vi "prep.vi"(8 "error in (no error)":errorcluster, 9 "Coordinate System":enum16{"Cartesian", "Cylindrical", "Spherical"}(ring), 10 "Plot processed data In":T1 caption="Data In", 11 "Parametric in":refnum<class "Parametric.lvclass">) -> (0 "error out":errorcluster, 2 "Plot Processed Data Out":T1 caption="Data Out", 3 "Parametric out":refnum<class "Parametric.lvclass">)   [LabVIEW 2017, in "Parametric.lvclass"]
uses:
  <vilib>/Native 3D Graph/classes/Parametric/Parametric.lvclass
  <vilib>/Native 3D Graph/xcontrol/Processed Data.ctl
  <vilib>/Native 3D Graph/typedefs/plot_rep_array.ctl
  <vilib>/Native 3D Graph/typedefs/plot_rep.ctl
  <vilib>/Native 3D Graph/typedefs/range_cluster.ctl
  <vilib>/Native 3D Graph/typedefs/min_max.ctl
  <vilib>/Native 3D Graph/typedefs/plot_rep_mesh_data.ctl
  <vilib>/Native 3D Graph/classes/Parametric/Parametric.lvclass/Parametric.ctl
  <vilib>/Analysis/coordinate.llb/3D Coordinate Conversion (Scalar).vi
  <vilib>/Native 3D Graph/classes/Base Datatype.lvclass
  <vilib>/Native 3D Graph/xcontrol/3DPC_SurfacePlot.xctl
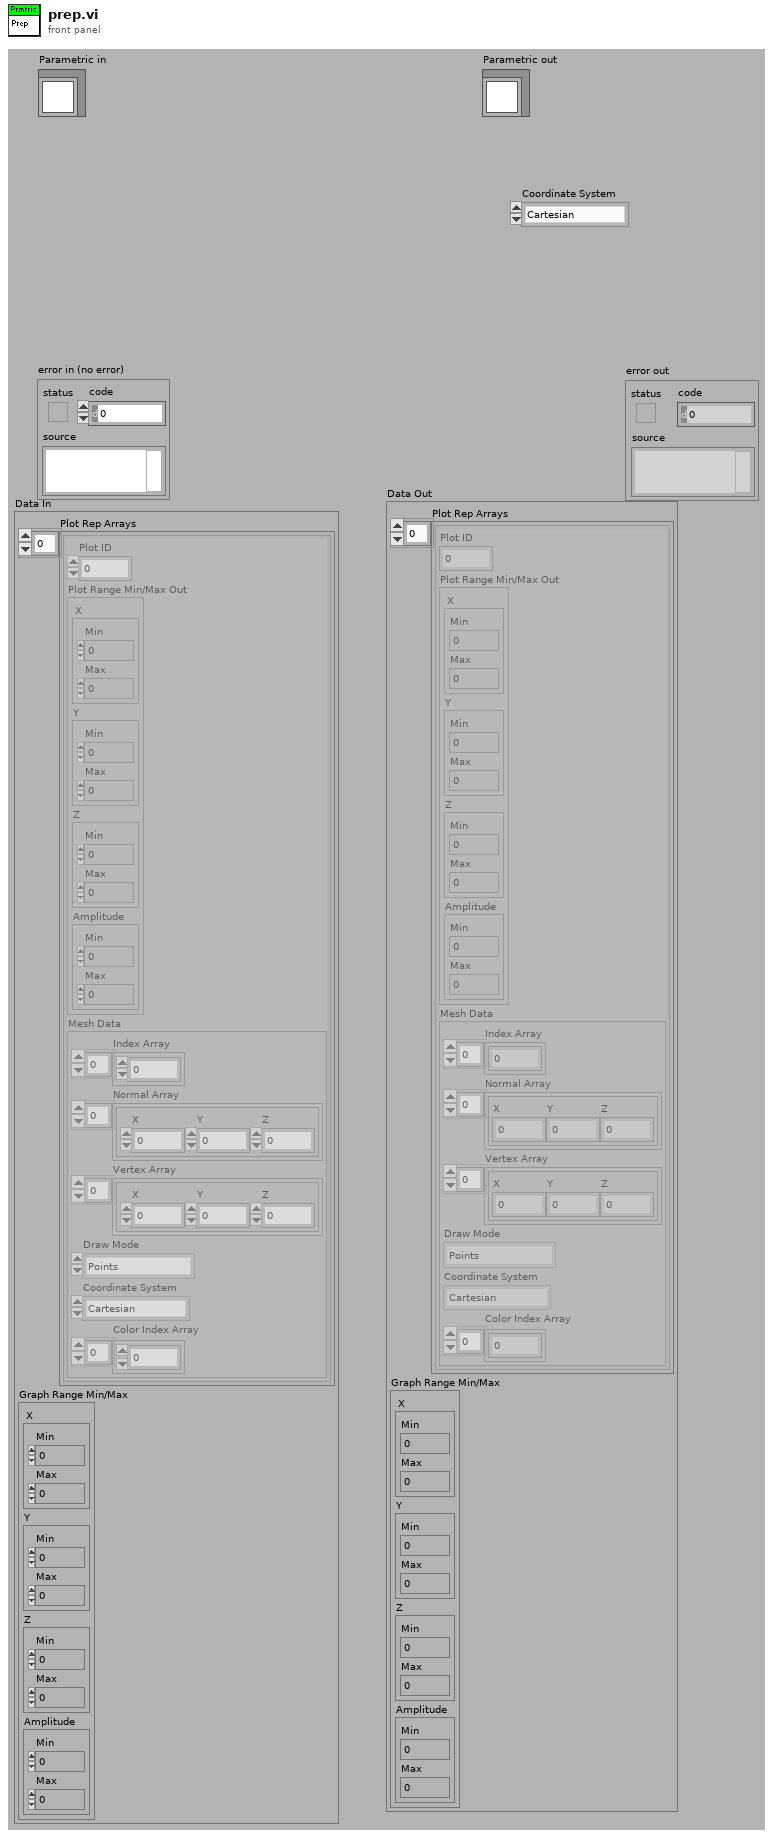
[diagram p1: front panel]
types:
  T1 = typedef "Processed Data.ctl" = cluster{"Plot Rep Arrays":T2, "Graph Range Min/Max":T4}
  T2 = typedef "3DPC_SurfacePlot.xctl/plot_rep_array.ctl" = T3[]
  T3 = typedef "3DPC_SurfacePlot.xctl/plot_rep.ctl" = cluster{"Plot ID":i32, "Plot Range Min/Max Out":T4, "Mesh Data":T6}
  T4 = typedef "3DPC_SurfacePlot.xctl/range_cluster.ctl" = cluster{"X":T5, "Y":T5, "Z":T5, "Amplitude":T5}
  T5 = typedef "3DPC_SurfacePlot.xctl/min_max.ctl" = cluster{"Min":sgl, "Max":sgl}
  T6 = typedef "3DPC_SurfacePlot.xctl/plot_rep_mesh_data.ctl" = cluster{"Index Array":u32[], "Normal Array":cluster{"X":sgl, "Y":sgl, "Z":sgl}[], "Vertex Array":cluster{"X":sgl, "Y":sgl, "Z":sgl}[], "Draw Mode":enum16{"Points", "Lines", "Line Strip", "Line Loop", "Triangles", "Triangle Strip", "Triangle Fan", "Quads", "Quad Strip", "Polygon"}, "Coordinate System":enum16{"Cartesian", "Cylindrical", "Spherical"}, "Color Index Array":i32[]}
  T7 = enum16{"Points", "Lines", "Line Strip", "Line Loop", "Triangles", "Triangle Strip", "Triangle Fan", "Quads", "Quad Strip", "Polygon"}
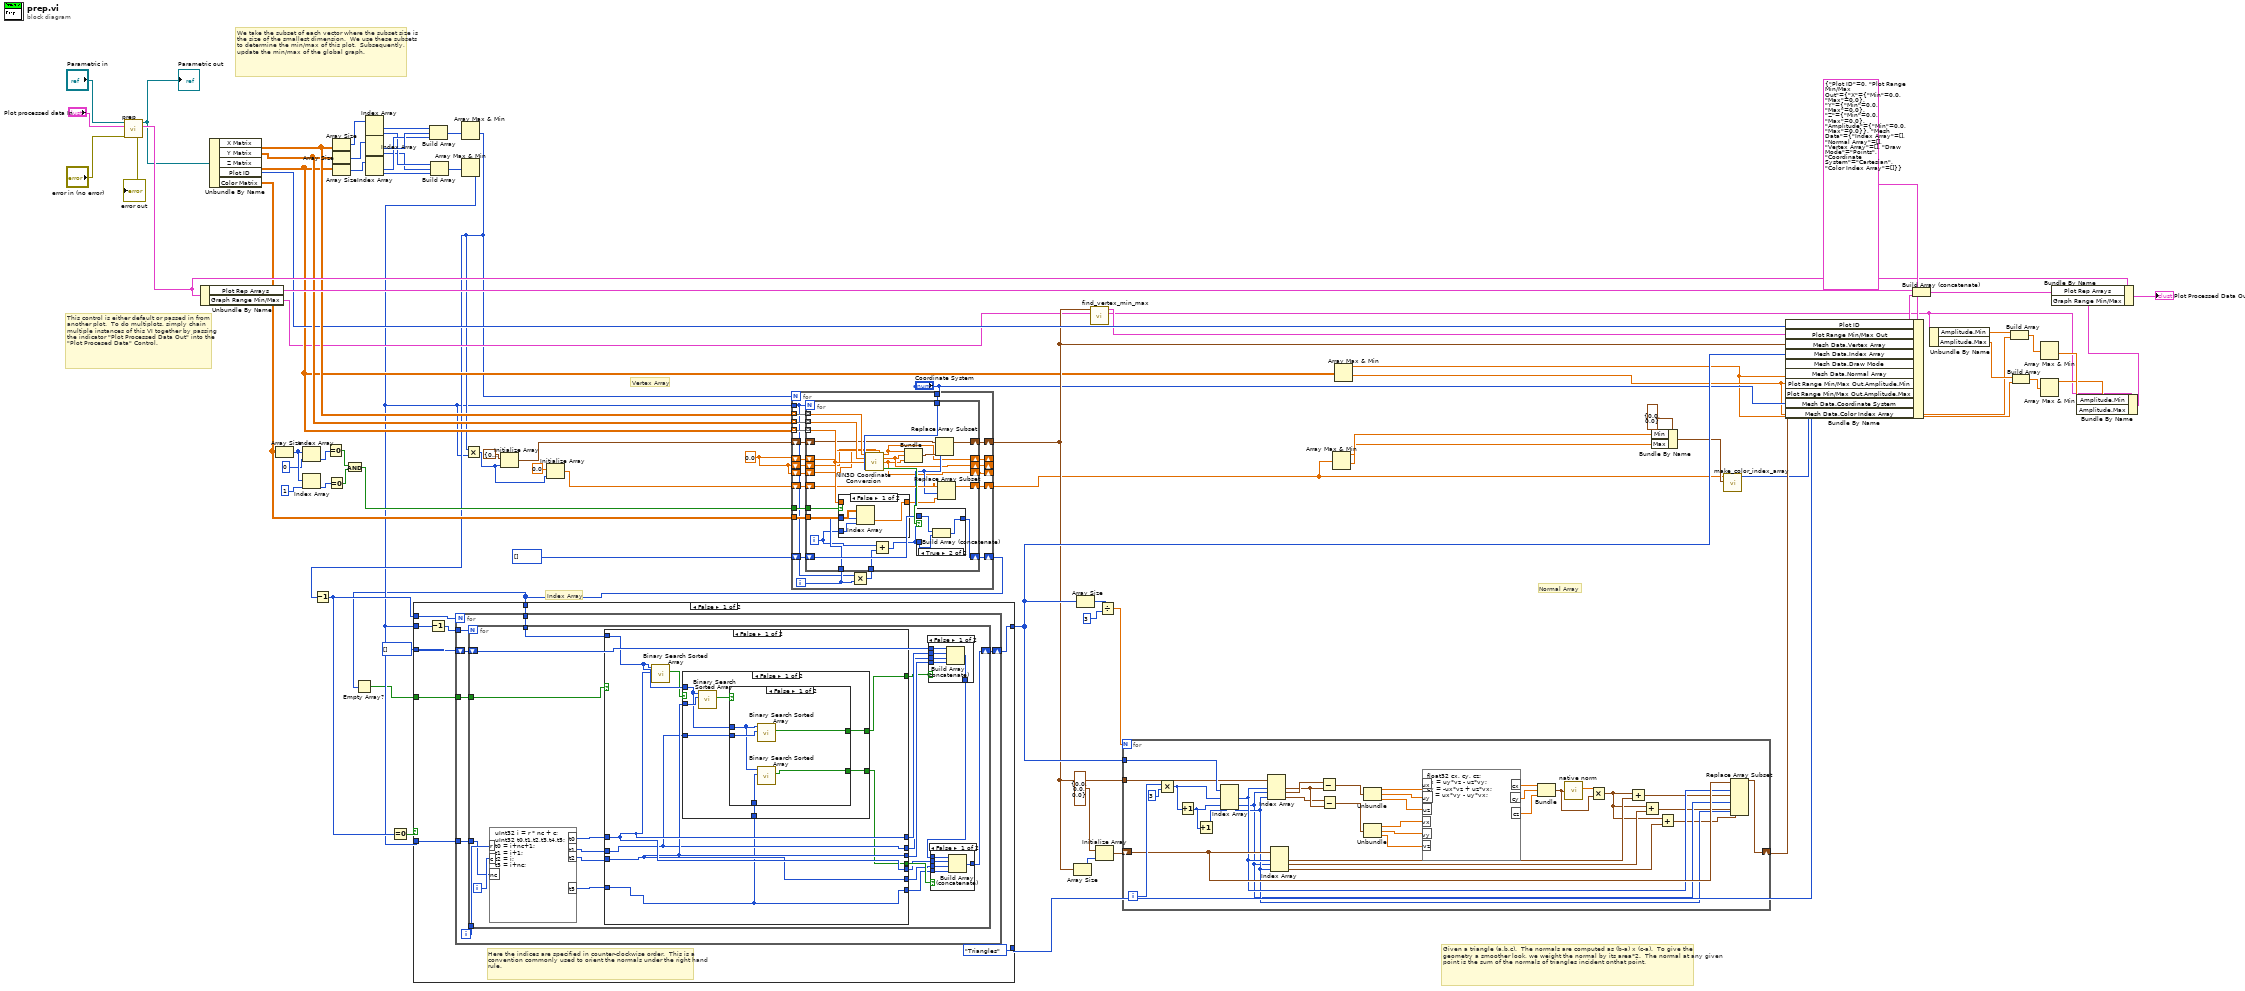
[diagram p0: block diagram]
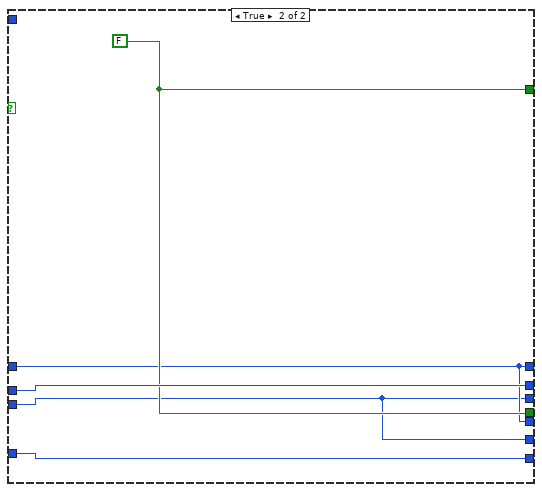
[diagram p6: hidden frame]
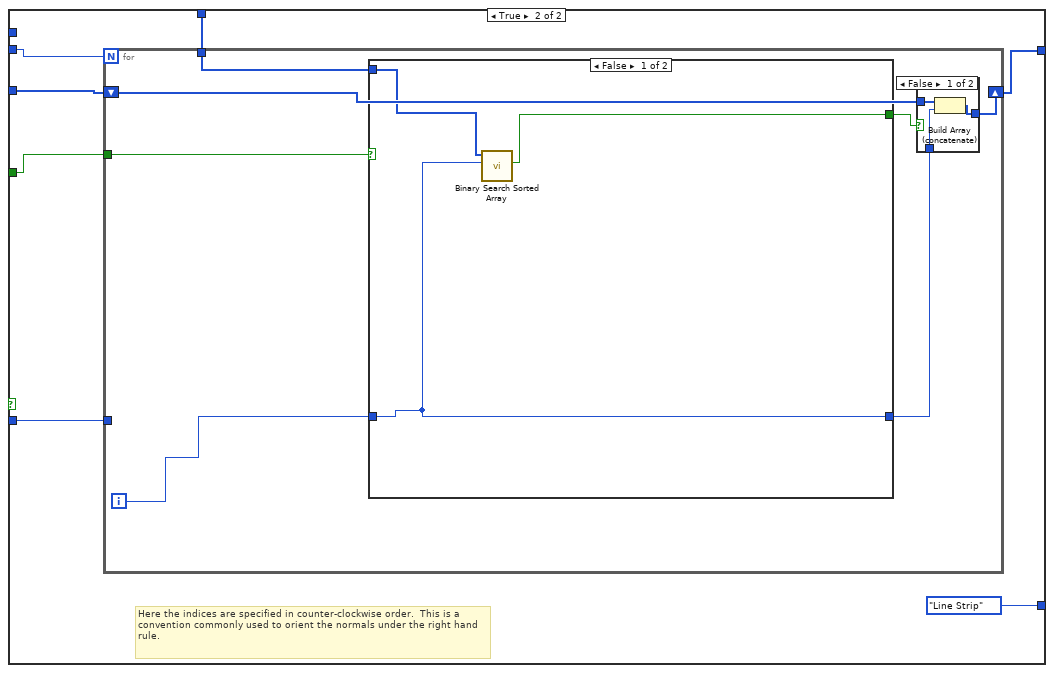
[diagram p7: hidden frame]
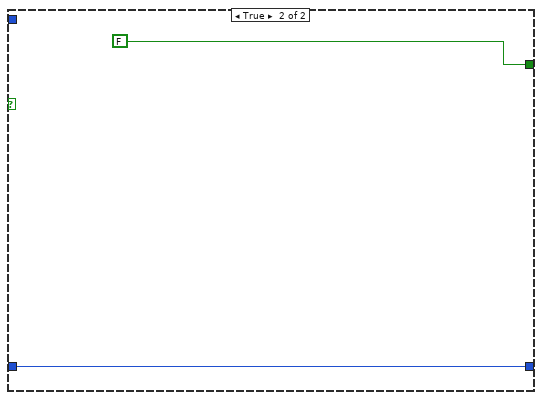
[diagram p9: hidden frame]
diagram:
  w3 = sgl 0.0
  # "Given a triangle (a,b,c).  The normals are computed as (b-a) x (c-a).  To give the geometry a smoother look, we weight the normal by its area*2.  The normal at any given point is the sum of the normals of triangles incident onthat point."
  # "Normal Array"
  # "Index Array"
  # "We take the subset of each vector where the subset size is the size of the smallest dimension.  We use these subsets to determine the min/max of this plot.  Subsequently, update the min/max of the global graph."
  # "This control is either default or passed in from another plot.  To do multiplots, simply chain multiple instances of this VI together by passing the indicator \"Plot Processed Data Out\" into the \"Plot Procesed Data\" Control."
  # "Vertex Array"
  n1 = call-parent "prep.vi"("error in (no error)"="error in (no error)", "Plot processed data In"="Plot processed data In", "Base Datatype in"="Parametric in") -> ("error out"=→"error out":errorcluster, "Plot processed Data Out"=w49:T1, "Base Datatype out"=w48:refnum<class "Parametric.lvclass">)  [unwired: 1 in, 5 out]
  "Parametric out" <- w48
  n2 = Unbundle By Name(w49) -> ("Plot Rep Arrays"=w73:T2, "Graph Range Min/Max"=w41:T4)
  n3 = Unbundle By Name(w48) -> ("X Matrix"=w47:sgl[][], "Y Matrix"=w46:sgl[][], "Z Matrix"=w42:sgl[][], "Plot ID"=w45:i32, "Color Matrix"=w20:sgl[][])
  n4 = Array Size(array=w20) -> (size(s)=w26:i32[])
  n5 = Index Array(array=w26, index=0) -> (element=w27:i32)
  n6 = Index Array(array=w26, index=1) -> (element=w28:i32)
  n7 = Equal To 0?(x=w27) -> (x = 0?=w23:bool)
  n8 = Equal To 0?(x=w28) -> (x = 0?=w22:bool)
  n9 = Array Size(array=w47) -> (size(s)=w69:i32[])
  n10 = Array Size(array=w46) -> (size(s)=w68:i32[])
  n11 = Array Size(array=w42) -> (size(s)=w67:i32[])
  n12 = And(x=w23, y=w22) -> (x .and. y?=w21:bool)
  n13 = Index Array(array=w69) -> (element #1=w66:i32, element #2=w63:i32)  [unwired: 2 in]
  n14 = Index Array(array=w68) -> (element #1=w65:i32, element #2=w62:i32)  [unwired: 2 in]
  n15 = Index Array(array=w67) -> (element #1=w64:i32, element #2=w61:i32)  [unwired: 2 in]
  n16 = Build Array(w66, w65, w64) -> (w60:i32[])
  n17 = Build Array(w63, w62, w61) -> (w59:i32[])
  n18 = Array Max & Min(array=w60) -> (min value=w10:i32)  [unwired: 3 out]
  n19 = Decrement(x=w10) -> (x-1=w14:i32)
  n20 = Equal To 0?(x=w14) -> (x = 0?=w13:bool)
  n21 = Array Max & Min(array=w59) -> (min value=w9:i32)  [unwired: 3 out]
  n22 = Multiply(x=w10, y=w9) -> (x*y=w5:i32)
  n23 = Initialize Array(cluster{"X":sgl, "Y":sgl, "Z":sgl} {"X"=0.0, "Y"=0.0, "Z"=0.0} ("3D Point"), w5) -> (w7:cluster{"X":sgl, "Y":sgl, "Z":sgl}[])
  n24 = Initialize Array(sgl 0.0, w5) -> (w4:sgl[])
  n25 = for {
    N: w10 -> [_]
    tunnel: w47 -> [w99] mode=indexing
    tunnel: w46 -> [w98] mode=indexing
    tunnel: w42 -> [w97] mode=indexing
    tunnel: w9 -> [w86]
    shift-right: [w95] -> w44
    shift-left: w7 -> [w96]
    tunnel: "Coordinate System" -> [w94]
    shift-right: [w92] -> w18
    shift-left: w4 -> [w93]
    tunnel: w21 -> [w91]
    tunnel: w20 -> [w90]
    shift-right: [w88] -> w2
    shift-left: u32[] [] -> [w89]
    shift-right: [w81] -> _
    shift-left: w3 -> [w84]
    shift-right: [w80] -> _
    shift-left: w3 -> [w83]
    shift-right: [w79] -> _
    shift-left: w3 -> [w82]
    i -> [w87]
    n26 = Multiply(x=w86, y=w87) -> (x*y=w85:i32)
    n27 = for {
      N: w86 -> [_]
      shift-right: [w111] -> w95
      shift-left: w96 -> [w112]
      tunnel: w99 -> [w122] mode=indexing
      tunnel: w98 -> [w123] mode=indexing
      tunnel: w97 -> [w120] mode=indexing
      tunnel: w94 -> [w124]
      shift-right: [w108] -> w92
      shift-left: w93 -> [w109]
      tunnel: w91 -> [w121]
      tunnel: w90 -> [w119]
      tunnel: w87 -> [w115]
      shift-right: [w116] -> w88
      shift-left: w89 -> [w117]
      tunnel: w85 -> [w114]
      shift-right: [w102] -> w81
      shift-left: w84 -> [w105]
      shift-right: [w101] -> w80
      shift-left: w83 -> [w104]
      shift-right: [w100] -> w79
      shift-left: w82 -> [w103]
      i -> [w113]
      n28 = case shown="False" w121 {
        tunnel: w120 -> [_ w133]
        tunnel: [w129 w133] -> w106
        tunnel: w119 -> [w132 _]
        tunnel: w115 -> [w131 _]
        tunnel: w113 -> [w130 _]
        frame False {
          n29 = Index Array(array=w132, index (row)=w131, index (col)=w130) -> (element=w129:sgl)
        }
        frame True {
        }
      }
      n30 = call <vilib>:"NIN3D Coordinate Conversion.vi"("X"=w122, "Z_prev"=w103, "Y_prev"=w104, "X_prev"=w105, "Y"=w123, "Z"=w120, "Coordinate System"=w124) -> ("X out"=w102:sgl, "Y out"=w101:sgl, "Z out"=w100:sgl, "NaN?"=w118:bool)  [unwired: 5 in]
      n31 = Add(x=w113, y=w114) -> (x+y=w107:i32)
      n32 = Bundle("X out"=w102, "Y out"=w101, "Z out"=w100) -> (w110:cluster{"X out":sgl, "Y out":sgl, "Z out":sgl})  [unwired: 1 out]
      n33 = case shown="True" w118 {
        tunnel: w117 -> [w125 w128]
        tunnel: [w125 w127] -> w116
        tunnel: w107 -> [_ w126]
        frame False {
        }
        frame True {
          n34 = Build Array (concatenate)(w128, w126) -> (w127:u32[])
        }
      }
      n35 = Replace Array Subset(array=w112, new element=w110, index=w107) -> (w111:cluster{"X":sgl, "Y":sgl, "Z":sgl}[])
      n36 = Replace Array Subset(array=w109, new element=w106, index=w107) -> (w108:sgl[])
    }
  }
  n37 = Empty Array?(array=w2) -> (empty?=w1:bool)
  n38 = case shown="False" w13 {
    tunnel: u32[] [] ("Indices") -> [w134 w215]
    tunnel: w9 -> [w142 w214]
    tunnel: [w141 w213] -> w51
    tunnel: w14 -> [w140 _]
    tunnel: w2 -> [w139 w212]
    tunnel: w9 -> [w138 w211]
    tunnel: [T7."Triangles" ("Mesh Data.Draw Mode") T7."Line Strip" ("Mesh Data.Draw Mode")] -> w11
    tunnel: w1 -> [w135 w209]
    frame False {
      # "Here the indices are specified in counter-clockwise order.  This is a convention commonly used to orient the normals under the right hand rule."
      n39 = Decrement(x=w138) -> (x-1=w137:i32)
      n40 = for {
        N: w140 -> [_]
        shift-right: [w145] -> w141
        shift-left: w134 -> [w149]
        tunnel: w137 -> [w147]
        tunnel: w142 -> [w146]
        tunnel: w139 -> [w144]
        tunnel: w135 -> [w143]
        i -> [w148]
        n41 = for {
          N: w147 -> [_]
          tunnel: w148 -> [w168]
          tunnel: w146 -> [w166]
          shift-right: [w154] -> w145
          shift-left: w149 -> [w169]
          tunnel: w144 -> [w161]
          tunnel: w143 -> [w150]
          i -> [w167]
          n42 = formula code="uInt32 i = r * nc + c; \nuInt32 t0,t1,t2,t3,t4,t5;\nt0 = i+nc+1; \nt1 = i+1; \nt2 = i; \nt5 = i+nc;"("r"=w168, "nc"=w166, "c"=w167) -> ("t0"=w165:u32, "t1"=w164:u32, "t2"=w163:u32, "t5"=w162:u32)
          n43 = case shown="False" w150 {
            tunnel: w161 -> [w189 _]
            tunnel: w165 -> [w188 w205]
            tunnel: [w188 w205] -> w160
            tunnel: w164 -> [w184 w208]
            tunnel: [w184 w208] -> w159
            tunnel: w163 -> [w185 w204]
            tunnel: [w185 w204] -> w158
            tunnel: [w188 w205] -> w153
            tunnel: [w185 w204] -> w152
            tunnel: w162 -> [w183 w207]
            tunnel: [w183 w207] -> w151
            tunnel: [w187 w206] -> w157
            tunnel: [w182 w206] -> w156
            frame False {
              n44 = call <vilib>:"Binary Search Sorted Array.vi"("Element"=w188, "Sorted Array"=w189) -> ("Found?"=w186:bool)  [unwired: 9 in]
              n45 = case shown="False" w186 {
                selector: w186 -> [_ w203]
                tunnel: w189 -> [w194 _]
                tunnel: w185 -> [w196 _]
                tunnel: [w193 w203] -> w187
                tunnel: w184 -> [w192 _]
                tunnel: w183 -> [w191 _]
                tunnel: [w190 w203] -> w182
                frame False {
                  n46 = call <vilib>:"Binary Search Sorted Array.vi"("Element"=w196, "Sorted Array"=w194) -> ("Found?"=w195:bool)  [unwired: 9 in]
                  n47 = case shown="False" w195 {
                    selector: w195 -> [_ w202]
                    tunnel: w194 -> [w198 _]
                    tunnel: w192 -> [w201 _]
                    tunnel: [w200 w202] -> w193
                    tunnel: w191 -> [w199 _]
                    tunnel: [w197 w202] -> w190
                    frame False {
                      n48 = call <vilib>:"Binary Search Sorted Array.vi"("Element"=w201, "Sorted Array"=w198) -> ("Found?"=w200:bool)  [unwired: 9 in]
                      n49 = call <vilib>:"Binary Search Sorted Array.vi"("Element"=w199, "Sorted Array"=w198) -> ("Found?"=w197:bool)  [unwired: 9 in]
                    }
                    frame True {
                    }
                  }
                }
                frame True {
                }
              }
            }
            frame True {
              w206 = FALSE
            }
          }
          n50 = case shown="False" w157 {
            tunnel: w169 -> [w180 w181]
            tunnel: w160 -> [w179 _]
            tunnel: w159 -> [w178 _]
            tunnel: w158 -> [w177 _]
            tunnel: [w176 w181] -> w155
            frame False {
              n51 = Build Array (concatenate)(w180, w179, w178, w177) -> (w176:u32[])
            }
            frame True {
            }
          }
          n52 = case shown="False" w156 {
            tunnel: w155 -> [w174 w175]
            tunnel: [w173 w175] -> w154
            tunnel: w153 -> [w172 _]
            tunnel: w152 -> [w171 _]
            tunnel: w151 -> [w170 _]
            frame False {
              n53 = Build Array (concatenate)(w174, w172, w171, w170) -> (w173:u32[])
            }
            frame True {
            }
          }
        }
      }
    }
    frame True {
      # "Here the indices are specified in counter-clockwise order.  This is a convention commonly used to orient the normals under the right hand rule."
      n54 = for {
        N: w211 -> [_]
        tunnel: w214 -> [_]
        shift-right: [w221] -> w213
        shift-left: w215 -> [w222]
        tunnel: w212 -> [w220]
        tunnel: w209 -> [w216]
        i -> [w217]
        n55 = case shown="False" w216 {
          tunnel: w220 -> [w229 _]
          tunnel: w217 -> [w228 w230]
          tunnel: [w227 FALSE] -> w219
          tunnel: [w228 w230] -> w218
          frame False {
            n56 = call <vilib>:"Binary Search Sorted Array.vi"("Element"=w228, "Sorted Array"=w229) -> ("Found?"=w227:bool)  [unwired: 9 in]
          }
          frame True {
          }
        }
        n57 = case shown="False" w219 {
          tunnel: w222 -> [w225 w226]
          tunnel: [w224 w226] -> w221
          tunnel: w218 -> [w223 _]
          frame False {
            n58 = Build Array (concatenate)(w225, w223) -> (w224:u32[])
          }
          frame True {
          }
        }
      }
    }
  }
  n59 = Array Size(array=w44) -> (size(s)=w57:i32)
  n60 = Array Size(array=w51) -> (size(s)=w53:i32)
  n61 = call <vilib>:"find_vertex_min_max.vi"("Total Range Min/Max"=w41, "Vertex Array"=w44) -> ("Total Range Out"=w32:T4, "This Range Min/Max Out"=w43:T4)  [unwired: 8 out]
  n62 = Initialize Array(cluster{"X":sgl, "Y":sgl, "Z":sgl} {"X"=0.0, "Y"=0.0, "Z"=0.0} ("3D Point"), w57) -> (w56:cluster{"X":sgl, "Y":sgl, "Z":sgl}[])
  n63 = Divide(x=w53, y=3) -> (x/y=w54:dbl)
  n64 = for {
    N: w54 -> [_]
    shift-right: [w258] -> w50
    shift-left: w56 -> [w261]
    tunnel: w51 -> [w264]
    tunnel: w44 -> [w256]
    i -> [w266]
    n65 = Multiply(x=w266, y=3) -> (x*y=w263:i32)
    n66 = Increment(x=w263) -> (x+1=w257:i32)
    n67 = Increment(x=w257) -> (x+1=w262:i32)
    n68 = Index Array(array=w264, index #1=w263, index #2=w257, index #3=w262) -> (element #1=w260:u32, element #2=w255:u32, element #3=w259:u32)
    n69 = Index Array(array=w256, index #1=w260, index #2=w255, index #3=w259) -> (element #1=w253:cluster{"X":sgl, "Y":sgl, "Z":sgl}, element #2=w254:cluster{"X":sgl, "Y":sgl, "Z":sgl}, element #3=w246:cluster{"X":sgl, "Y":sgl, "Z":sgl})
    n70 = Index Array(array=w261, index #1=w260, index #2=w255, index #3=w259) -> (element #1=w252:cluster{"X":sgl, "Y":sgl, "Z":sgl}, element #2=w251:cluster{"X":sgl, "Y":sgl, "Z":sgl}, element #3=w249:cluster{"X":sgl, "Y":sgl, "Z":sgl})
    n71 = Subtract(x=w254, y=w253) -> (x-y=w234:cluster{"X":sgl, "Y":sgl, "Z":sgl})
    n72 = Subtract(x=w246, y=w253) -> (x-y=w233:cluster{"X":sgl, "Y":sgl, "Z":sgl})
    n73 = Unbundle(w234) -> ("X"=w243:sgl, "Y"=w242:sgl, "Z"=w241:sgl)
    n74 = Unbundle(w233) -> ("X"=w240:sgl, "Y"=w239:sgl, "Z"=w238:sgl)
    n75 = formula code="float32 cx, cy, cz;\ncx = uy*vz - uz*vy;\ncy = -ux*vz + uz*vx;\ncz = ux*vy - uy*vx;"("ux"=w243, "uy"=w242, "uz"=w241, "vx"=w240, "vy"=w239, "vz"=w238) -> ("cx"=w237:sgl, "cy"=w236:sgl, "cz"=w235:sgl)
    n76 = Bundle(w237, w236, w235) -> (w232:cluster{sgl, sgl, sgl})  [unwired: 1 out]
    n77 = call <vilib>:"native norm.vi"("Vector"=w232) -> ("Norm"=w244:sgl)  [unwired: 10 in]
    n78 = Multiply(x=w244, y=w232) -> (x*y=w250:cluster{sgl, sgl, sgl})
    n79 = Add(x=w250, y=w252) -> (x+y=w245:cluster{sgl, sgl, sgl})
    n80 = Add(x=w250, y=w251) -> (x+y=w248:cluster{sgl, sgl, sgl})
    n81 = Add(x=w250, y=w249) -> (x+y=w247:cluster{sgl, sgl, sgl})
    n82 = Replace Array Subset(array=w261, new element #1=w245, index #1=w260, new element #2=w248, index #2=w255, new element #3=w247, index #3=w259) -> (w258:cluster{"X":sgl, "Y":sgl, "Z":sgl}[])
  }
  n83 = Array Max & Min(array=w18) -> (max value=w15:sgl, min value=w16:sgl)  [unwired: 2 out]
  n84 = Array Max & Min(array=w42) -> (max value=w17:sgl, min value=w19:sgl)  [unwired: 2 out]
  n85 = Bundle By Name(cluster=T5 {"Min"=0.0, "Max"=0.0} ("Amplitude"), "Min"=w16, "Max"=w15) -> (w30:T5)
  n86 = call <vilib>:"make_color_index_array.vi"("Amplitude Min/Max"=w30, "Z array"=w18) -> ("Color Index Array"=w29:i32[])  [unwired: 9 out]
  n87 = Bundle By Name(cluster=T3 {"Plot ID"=0, "Plot Range Min/Max Out"={"X"={"Min"=0.0, "Max"=0.0}, "Y"={"Min"=0.0, "Max"=0.0}, "Z"={"Min"=0.0, "Max"=0.0}, "Amplitude"={"Min"=0.0, "Max"=0.0}}, "Mesh Data"={"Index Array"=[], "Normal Array"=[], "Vertex Array"=[], "Draw Mode"=enum."Points", "Coordinate System"=enum."Cartesian", "Color Index Array"=[]}} ("Plot Representation"), "Plot ID"=w45, "Plot Range Min/Max Out"=w43, "Mesh Data.Vertex Array"=w44, "Mesh Data.Index Array"=w51, "Mesh Data.Draw Mode"=w11, "Mesh Data.Normal Array"=w50, "Plot Range Min/Max Out.Amplitude.Min"=w19, "Plot Range Min/Max Out.Amplitude.Max"=w17, "Mesh Data.Coordinate System"="Coordinate System", "Mesh Data.Color Index Array"=w29) -> (w72:T3)
  n88 = Build Array (concatenate)(w73, w72) -> (w71:T2)
  n89 = Unbundle By Name(w32) -> ("Amplitude.Min"=w39:sgl, "Amplitude.Max"=w36:sgl)
  n90 = Build Array(w39, w19) -> (w38:sgl[])
  n91 = Build Array(w36, w17) -> (w35:sgl[])
  n92 = Array Max & Min(array=w38) -> (min value=w37:sgl)  [unwired: 3 out]
  n93 = Array Max & Min(array=w35) -> (max value=w34:sgl)  [unwired: 3 out]
  n94 = Bundle By Name(cluster=w32, "Amplitude.Min"=w37, "Amplitude.Max"=w34) -> (w33:T4)
  n95 = Bundle By Name(cluster=w49, "Plot Rep Arrays"=w71, "Graph Range Min/Max"=w33) -> (→"Plot Processed Data Out":T1)
